vi "daqtest.vi"() -> ()   [LabVIEW 2013]
uses:
  <vilib>/DAQmx/write.llb/DAQmx Write (Analog Wfm 1Chan NSamp).vi
  <vilib>/DAQmx/create/channels.llb/DAQmx Create Channel (AO-Voltage-Basic).vi
  <vilib>/DAQmx/configure/trigger.llb/DAQmx Start Trigger (Digital Edge).vi
  <vilib>/DAQmx/configure/timing.llb/DAQmx Timing (Use Waveform).vi
  <vilib>/DAQmx/miscellaneous.llb/DAQmx Fill In Error Info.vi
panel:
  in  "wait time":dbl
  in  "End Voltage":dbl
  in  "Start Voltage":dbl
  in  "dt":dbl
  in  "ramp time":dbl
  in  "stop 2":bool
  in  "source":tag
  out "error out":errorcluster
  out "NumSampl/Chan":u32
  out "output waveform":waveform(dbl)(graph)
  in  "edge":i32(ring)=10280 items=["Rising"=10280, "Falling"=10171]
  in  "units":i32(ring)=10348 items=["Volts"=10348, "From Custom Scale"=10065]
  in  "Task Name":string
  in  "physical channels":tag
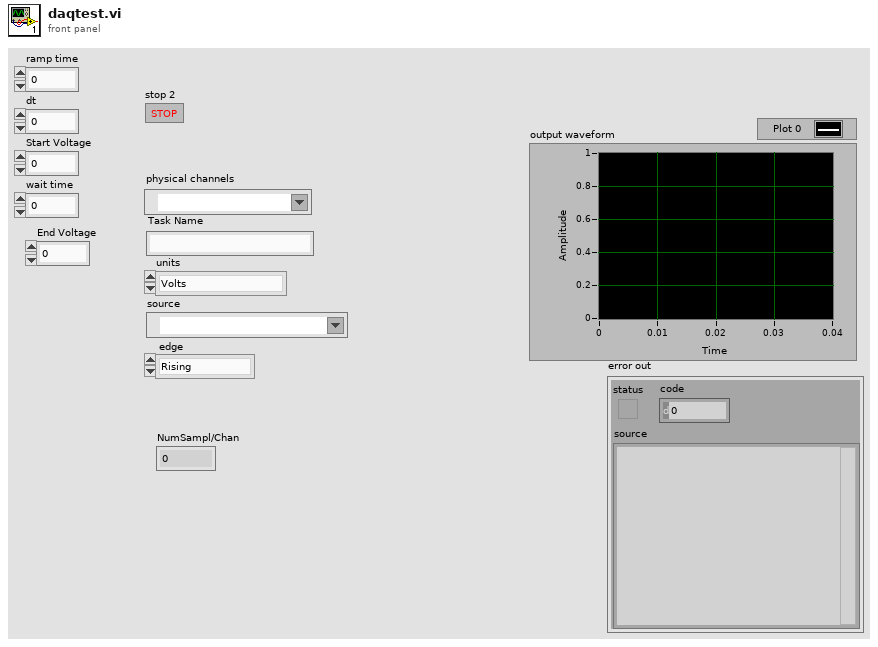
[diagram p1: front panel]
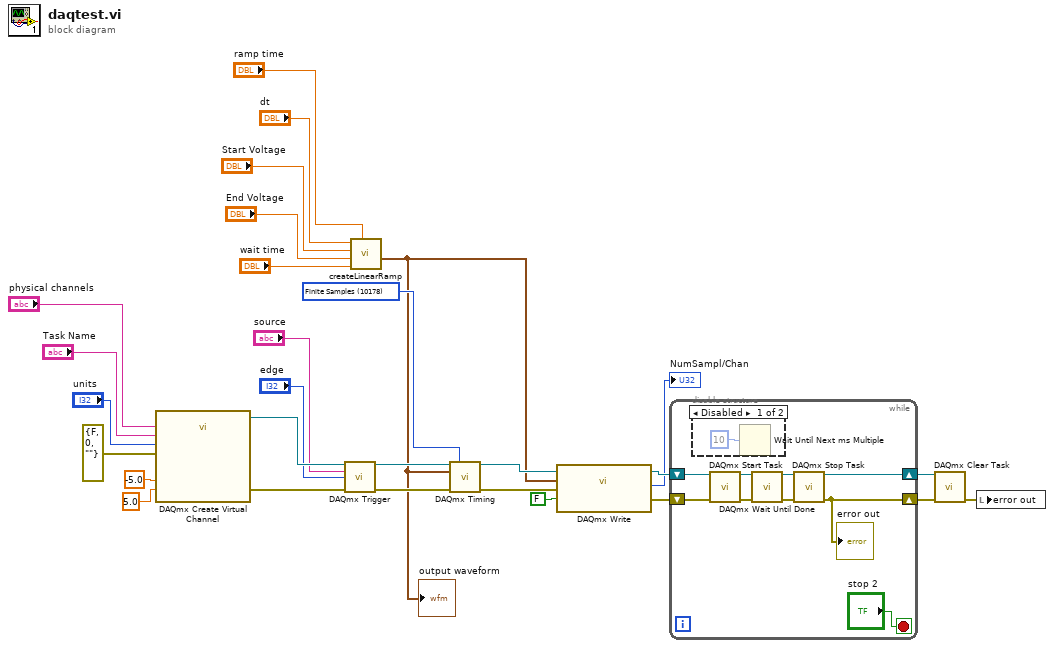
[diagram p0: block diagram]
diagram:
  w11 = 10178 items=["Finite Samples"=10178, "Continuous Samples"=10123, "Hardware Timed Single Point"=12522] ("sample mode")
  n1 = call-poly <vilib>:"DAQmx Create Virtual Channel.vi"("maximum value"=5.0, "minimum value"=-5.0, "physical channels"="physical channels", "name to assign"="Task Name", "units"="units", "error in"=errorcluster {"status"=FALSE, "code"=0, "source"=""}) -> ("task out"=w22:refnum<k21>, "error out"=w20:errorcluster)  [unwired: 8 in]
  n2 = call-poly <vilib>:"DAQmx Trigger.vi"("task/channels in"=w22, "source"="source", "edge"="edge", "error in"=w20) -> ("task out"=w14:refnum<k21>, "error out"=w13:errorcluster)  [unwired: 10 in]
  n3 = call "createLinearRamp.vi"("ramp time"="ramp time", "wait time"="wait time", "End Voltage"="End Voltage", "Start Voltage"="Start Voltage", "dt"="dt") -> ("output waveform"=w6:waveform(dbl))  [unwired: 6 in]
  "output waveform" <- w6
  n4 = call-poly <vilib>:"DAQmx Timing.vi"("task/channels in"=w14, "sample mode"=w11, "waveform"=w6, "error in"=w13) -> ("task out"=w7:refnum<k21>, "error out"=w8:errorcluster)  [unwired: 10 in]
  n5 = call-poly <vilib>:"DAQmx Write.vi"("task/channels in"=w7, "auto start"=FALSE, "data"=w6, "error in"=w8) -> ("task out"=w18:refnum<k21>, "number of samples written per channel"=→"NumSampl/Chan":u32, "error out"=w19:errorcluster)  [unwired: 9 in]
  n6 = while {
    shift-right: [w37] -> w16
    shift-left: w18 -> [w36]
    shift-right: [w33] -> w17
    shift-left: w19 -> [w35]
    stop <- "stop 2" stop-if-true
    n7 = disable-structure shown="Disabled" {
      frame Disabled {
        n8 = Wait Until Next ms Multiple(millisecond multiple=u32 10) -> ()  [unwired: 1 out]
      }
      frame Enabled {
      }
    }
    n9 = call <vilib>:"DAQmx Start Task.vi"("task/channels in"=w36, "error in"=w35) -> ("task out"=w30:refnum<k21>, "error out"=w29:errorcluster)  [unwired: 12 in]
    n10 = call <vilib>:"DAQmx Wait Until Done.vi"("task/channels in"=w30, "error in"=w29) -> ("task out"=w32:refnum<k21>, "error out"=w31:errorcluster)  [unwired: 12 in]
    n11 = call <vilib>:"DAQmx Stop Task.vi"("task/channels in"=w32, "error in"=w31) -> ("task out"=w37:refnum<k21>, "error out"=w33:errorcluster)  [unwired: 12 in]
    "error out" <- w33
  }
  n12 = call <vilib>:"DAQmx Clear Task.vi"("task in"=w16, "error in"=w17) -> ("error out"=w15:errorcluster)  [unwired: 13 in]
  n13 = local write "error out"(w15) -> ()
